vi "Set_Wavelength_Step.vi"(8 "error in (no error)":errorcluster, 10 "wave step":dbl, 11 ".NET Reference in":refnum<k24>) -> (0 "error out":errorcluster, 3 ".NET Reference out":refnum<k24>)   [LabVIEW 2017]
uses:
  C:/Users/Ssantec_Test/Documents/Instrument_DLL_Sample_Labview_20250826_Ver1.5.0_x64/DLL/InstrumentDLL.dll
  DLL/InstrumentDLL.dll
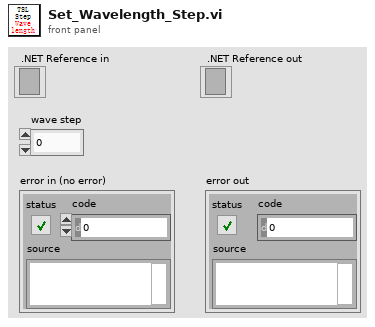
[diagram p1: front panel]
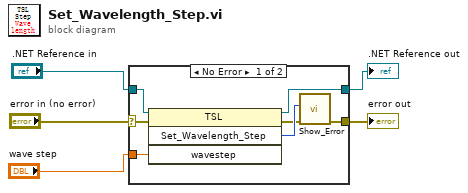
[diagram p0: block diagram]
diagram:
  n1 = case shown="No Error" "error in (no error)" {
    selector: "error in (no error)" -> [w6 w13]
    tunnel: "wave step" -> [w12 _]
    tunnel: [w7 w13] -> w4
    tunnel: [w11 w14] -> w3
    tunnel: ".NET Reference in" -> [w10 w14]
    frame No Error {
      n2 = invoke on="调用节点" class="TSL" method="Set_Wavelength_Step"(reference=w10, error in=w6, "wavestep"=w12) -> (reference out=w11:refnum<k24>, error out=w8:errorcluster, "Set_Wavelength_Step"=w9:i32)  [unwired: 1 in, 1 out]
      n3 = call "Show_Error.vi"("error in (no error)"=w8, "Error"=w9) -> ("error out"=w7:errorcluster)  [unwired: 9 in]
    }
    frame Error {
    }
  }
  "error out" <- w4
  ".NET Reference out" <- w3
